vi "Test Storage Panel Template TDMS.vi"(6 "Fields In":T1[](array[typedef]), 8 "error in (no error)":errorcluster, 10 "Test Results":string, 11 "TDMS File Ref":refnum<k34>) -> (0 "error out":errorcluster, 3 "TDMS File Ref":refnum<k34>, 4 "Fields Out":T1[](array[typedef]))   [LabVIEW 2011]
uses:
  server/database/Fields/Field Record.ctl
  server/database/Fields/Field DataTypes.ctl
  server/database/Fields/Field NextItem.ctl
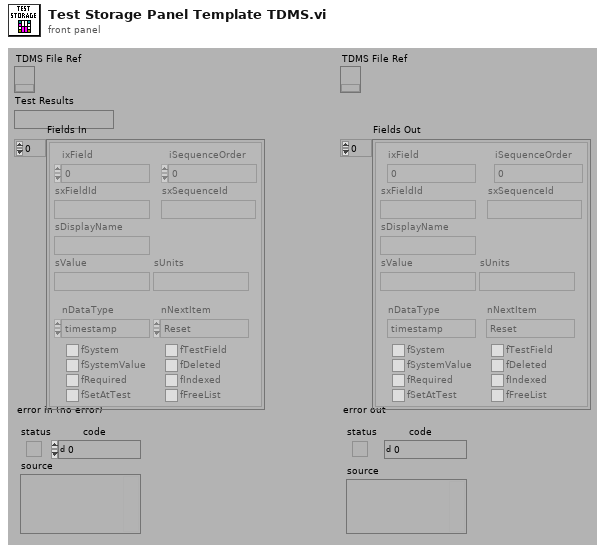
[diagram p1: front panel]
types:
  T1 = typedef "Field Record.ctl" = cluster{"ixField":i32, "iSequenceOrder":i32, "sxFieldId":string, "sxSequenceId":string, "sDisplayName":string, "sValue":string, "sUnits":string, "nDataType":T2, "nNextItem":T3, "fSystem":bool, "fSystemValue":bool, "fRequired":bool, "fSetAtTest":bool, "fTestField":bool, "fDeleted":bool, "fIndexed":bool, "fFreeList":bool}
  T2 = typedef "Field DataTypes.ctl" = enum32{"text", "numeric", "list", "timestamp", "boolean"}
  T3 = typedef "Field NextItem.ctl" = enum32{"Reset", "Retain", "Auto-Increment"}
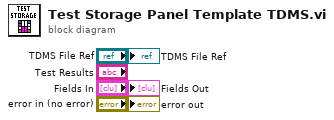
[diagram p0: block diagram]
diagram:
